vi "uManagerReadTXT.vi"(4 "numImg":u32, 5 "expTime":dbl, 6 "error in (no error)":errorcluster, 7 "start":dbl, 8 "file path labViewCom":path, 9 "file path AcqSettings":path) -> (0 "error out":errorcluster)   [LabVIEW 2021]
panel:
  out "AcqSettingsOut":string
  out "numImgDigg":string
  out "labViewComOut":string
  out "numImgDig":string
  out "expTimeDig":string
  out "startDig":string
  out "AcqSettings":string="Start: 1; ExpTime: 10; NumOfImages: 100;"
  out "labViewCom":string="Start: 1; ExpTime: 10; NumOfImages: 100;"
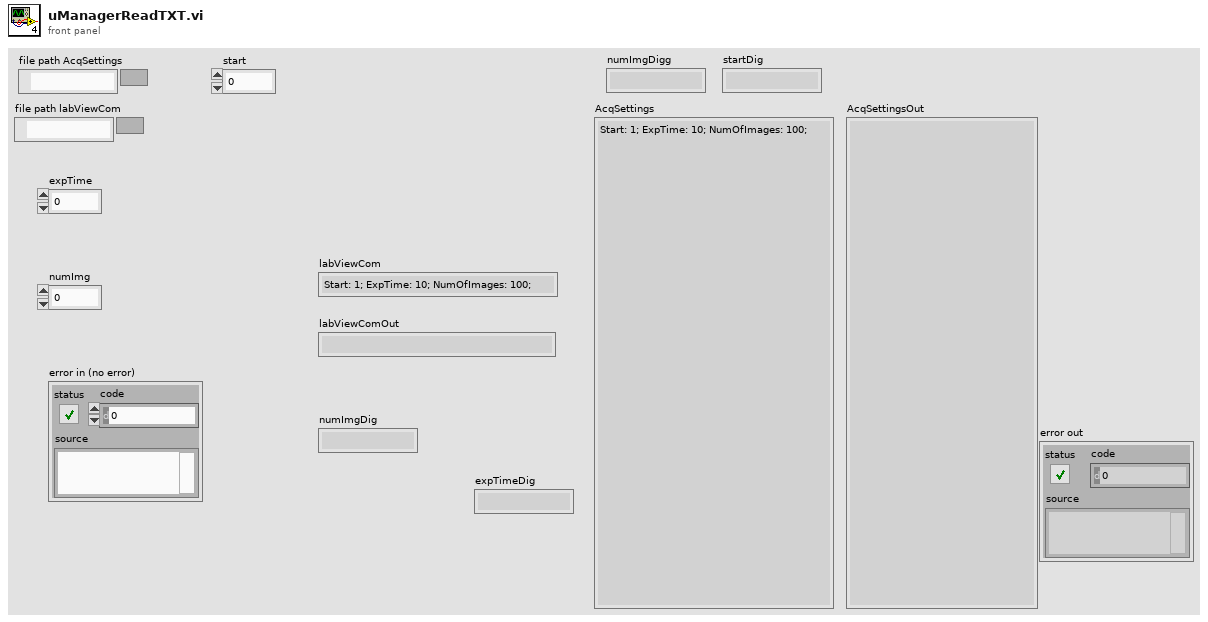
[diagram p1: front panel]
types:
  T1 = enum16{"open", "replace", "create", "open or create", "replace or create", "replace or create with confirmation"}
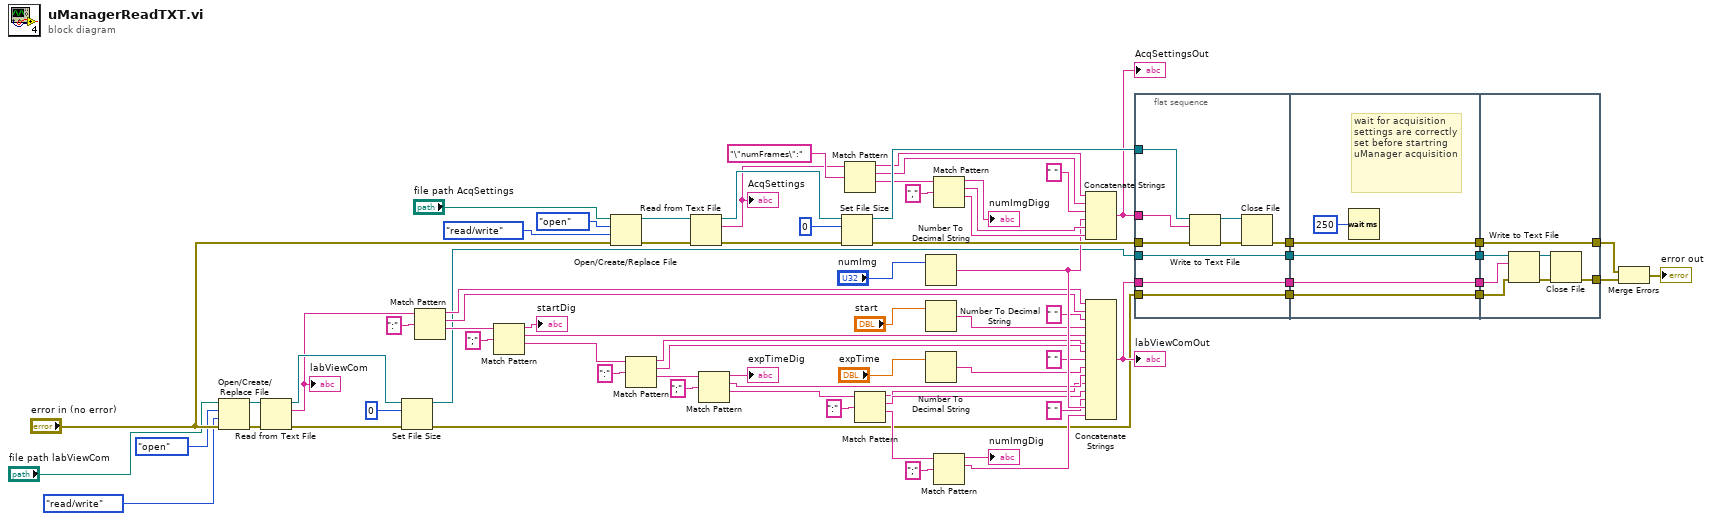
[diagram p0: block diagram]
diagram:
  n1 = Open/Create/Replace File(file path (use dialog)="file path labViewCom", error in="error in (no error)", operation (0:open)=T1."open", access (0:read/write)=enum16{"read/write", "read-only", "write-only"}."read/write") -> (refnum out=w17:refnum<file>, error out=w13:errorcluster)  [unwired: 2 in, 1 out]
  n2 = Read from Text File(file (use dialog)=w17, error in=w13) -> (refnum out=w69:refnum<file>, text=w37:string, error out=w68:errorcluster)  [unwired: 2 in, 1 out]
  "labViewCom" <- w37
  n3 = Set File Size(4:w68, 6:i64 0 ("offset (in bytes) (0)"), 7:w69) -> (0:w4:errorcluster, 3:w10:refnum<file>)
  n4 = Match Pattern(string=w37, regular expression=":") -> (before substring=w39:string, match substring=w40:string, after substring=w26:string)  [unwired: 1 in, 1 out]
  n5 = Match Pattern(string=w26, regular expression=";") -> (before substring=→"startDig":string, match substring=w53:string, after substring=w41:string)  [unwired: 1 in, 1 out]
  n6 = Open/Create/Replace File(file path (use dialog)="file path AcqSettings", error in="error in (no error)", operation (0:open)=T1."open", access (0:read/write)=enum16{"read/write", "read-only", "write-only"}."read/write") -> (refnum out=w22:refnum<file>, error out=w23:errorcluster)  [unwired: 2 in, 1 out]
  n7 = Match Pattern(string=w41, regular expression=":") -> (before substring=w44:string, match substring=w45:string, after substring=w31:string)  [unwired: 1 in, 1 out]
  n8 = Read from Text File(file (use dialog)=w22, error in=w23) -> (refnum out=w73:refnum<file>, text=w58:string, error out=w76:errorcluster)  [unwired: 2 in, 1 out]
  "AcqSettings" <- w58
  n9 = Match Pattern(string=w31, regular expression=";") -> (before substring=→"expTimeDig":string, match substring=w56:string, after substring=w38:string)  [unwired: 1 in, 1 out]
  n10 = Set File Size(4:w76, 6:i64 0 ("size (in bytes)"), 7:w73) -> (0:w77:errorcluster, 3:w74:refnum<file>)
  n11 = Match Pattern(string=w58, regular expression="\"numFrames\":") -> (before substring=w62:string, match substring=w63:string, after substring=w57:string)  [unwired: 1 in, 1 out]
  n12 = Match Pattern(string=w38, regular expression=":") -> (before substring=w48:string, match substring=w49:string, after substring=w34:string)  [unwired: 1 in, 1 out]
  n13 = Number To Decimal String(number="numImg") -> (decimal integer string=w64:string)  [unwired: 1 in]
  n14 = Number To Decimal String(number="start") -> (decimal integer string=w54:string)  [unwired: 1 in]
  n15 = Number To Decimal String(number="expTime") -> (decimal integer string=w55:string)  [unwired: 1 in]
  n16 = Match Pattern(string=w57, regular expression=",") -> (before substring=→"numImgDigg":string, match substring=w66:string, after substring=w67:string)  [unwired: 1 in, 1 out]
  n17 = Match Pattern(string=w34, regular expression=";") -> (before substring=→"numImgDig":string, match substring=w52:string)  [unwired: 1 in, 2 out]
  n18 = Concatenate Strings(w62, w63, " " ("string"), w64, w66, w67) -> (w71:string)
  "AcqSettingsOut" <- w71
  n19 = Concatenate Strings(w39, w40, " " ("string"), w54, w53, w44, w45, " " ("string"), w55, w56, w48, w49, " " ("string"), w64, w52) -> (w7:string)
  "labViewComOut" <- w7
  n20 = flat-sequence {
    tunnel: w77 -> [w86]
    tunnel: w74 -> [w85]
    tunnel: w71 -> [w84]
    tunnel: [w79] -> w12
    tunnel: w10 -> [w83]
    tunnel: [w83] -> w9
    tunnel: w7 -> [w82]
    tunnel: [w82] -> w5
    tunnel: w4 -> [w81]
    tunnel: [w81] -> w2
    tunnel: w12 -> [w91]
    tunnel: [w91] -> w11
    tunnel: w9 -> [w90]
    tunnel: [w90] -> w8
    tunnel: [w89] -> w6
    tunnel: w5 -> [w89]
    tunnel: [w88] -> w3
    tunnel: w2 -> [w88]
    tunnel: [w98] -> w72
    tunnel: w11 -> [w98]
    tunnel: w8 -> [w97]
    tunnel: w6 -> [w96]
    tunnel: w3 -> [w95]
    tunnel: [w92] -> w1
    frame #0 {
      n21 = Write to Text File(file (use dialog)=w85, text=w84, error in=w86) -> (refnum out=w78:refnum<file>, error out=w80:errorcluster)  [unwired: 1 in, 1 out]
      n22 = Close File(refnum=w78, error in=w80) -> (error out=w79:errorcluster)  [unwired: 1 out]
    }
    frame #1 {
      # "wait for acquisition settings are correctly set before startring uManager acquisition"
      n23 = Wait (ms)(milliseconds to wait=u32 250) -> ()  [unwired: 1 out]
    }
    frame #2 {
      n24 = Write to Text File(file (use dialog)=w97, text=w96, error in=w95) -> (refnum out=w94:refnum<file>, error out=w93:errorcluster)  [unwired: 1 in, 1 out]
      n25 = Close File(refnum=w94, error in=w93) -> (error out=w92:errorcluster)  [unwired: 1 out]
    }
  }
  n26 = Merge Errors(w72, w1) -> (→"error out":errorcluster)
